vi "setPressure_topLvl.vi"(5 "which manipulator":T1(ring), 7 "Slide Refnum":refnum<vi>, 8 "error in":errorcluster, 10 "set pressure (mBar)":dbl format="%#_13g", 11 "Pressure box control in":T2={"Pressure box COM"="COM7", "pressure box type"=enum."Neuromatics", "High pos pressure (mBar)"=200.0, "Low pos pressure (mBar)"=80.0, "Vacuum pressure (mBar)"=-40.0, "calibration"=enum."mightenRig"}) -> (0 "error out":errorcluster, 3 "Pressure box control out":T2={"Pressure box COM"="", "pressure box type"=enum."Neuromatics", "High pos pressure (mBar)"=200.0, "Low pos pressure (mBar)"=80.0, "Vacuum pressure (mBar)"=-40.0, "calibration"=enum."PA_vacPump"})   [LabVIEW 2019]
uses:
  controls/pressure_box_control.ctl
  controls/pressure_box_type.ctl
  controls/arduino_pressure_setting.ctl
  controls/proportionAir_cmds.ctl
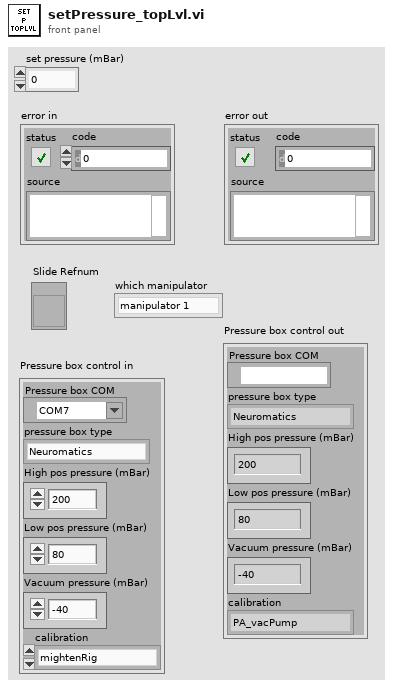
[diagram p1: front panel]
types:
  T1 = enum16{"manipulator 1", "manipulator 2", "manipulator 3", "manipulator 4"}
  T2 = typedef "pressure_box_control.ctl" = cluster{"Pressure box COM":refnum<visa-resource-name>, "pressure box type":T3, "High pos pressure (mBar)":dbl, "Low pos pressure (mBar)":dbl, "Vacuum pressure (mBar)":dbl, "calibration":enum16{"PA_vacPump", "PA_venturi", "Neuromatics", "ilyaRig", "mightenRig"}}
  T3 = typedef "pressure_box_type.ctl" = enum16{"Neuromatics", "ProportionAir", "Demo box", "N-ProportionAir"}
  T4 = enum16{"PA_vacPump", "PA_venturi", "Neuromatics", "ilyaRig", "mightenRig"}
  T5 = typedef "arduino_pressure_setting.ctl" = enum16{"High Positive Pressure", "Low Positive Pressure", "Atmospheric Pressure", "Low Vacuum", "High Vacuum", "Break In", "Puff"}
  T6 = typedef "proportionAir_cmds.ctl" = enum16{"Set P", "Switch to Atm", "Switch to Regulator", "Pulse", "WC"}
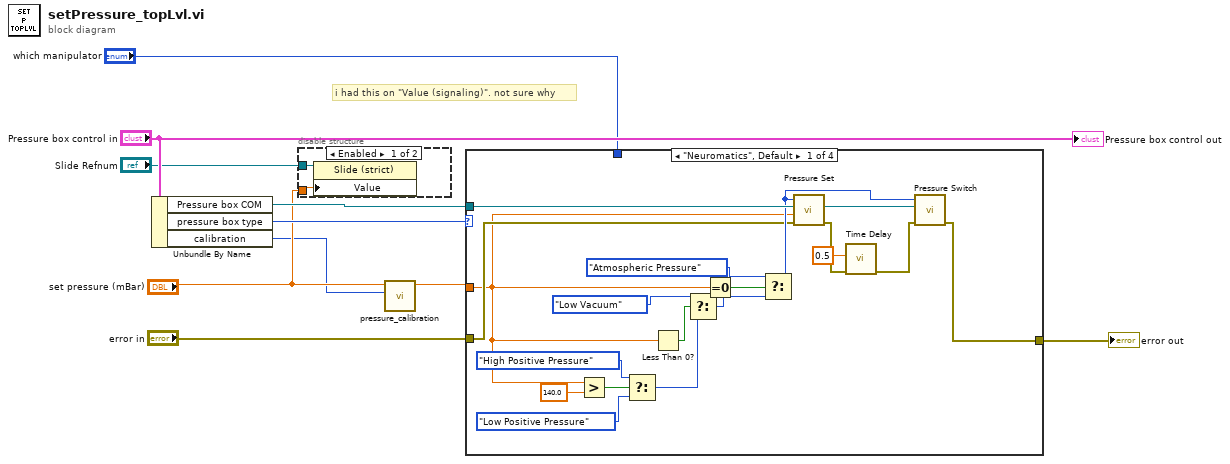
[diagram p0: block diagram]
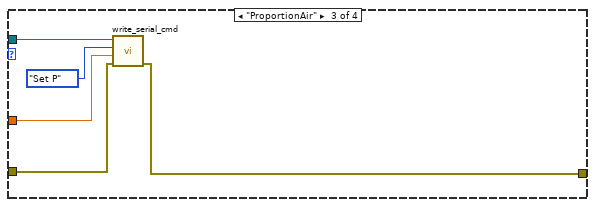
[diagram p4: hidden frame]
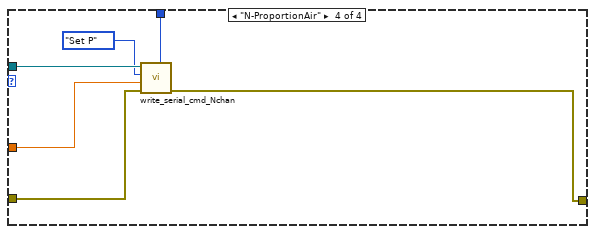
[diagram p5: hidden frame]
diagram:
  # "i had this on \"Value (signaling)\". not sure why"
  n1 = Unbundle By Name("Pressure box control in") -> ("Pressure box COM"=w9:refnum<visa-resource-name>, "pressure box type"=w10:T3, "calibration"=w1:T4)
  n2 = disable-structure shown="Enabled" {
    disable-tunnel: "Slide Refnum" -> [w12 _]
    disable-tunnel: "set pressure (mBar)" -> [w11 _]
    frame Enabled {
      n3 = property class="Slide (strict)"(reference=w12, "Value"=w11) -> ()  [unwired: 1 in, 2 out]
    }
    frame Disabled {
    }
  }
  n4 = call "pressure_calibration.vi"("calibration"=w1, "cmd pressure (mBar)"="set pressure (mBar)") -> ("pressure out (mbar)"=w5:dbl)  [unwired: 9 in]
  n5 = case shown="\"Neuromatics\", Default" w10 {
    tunnel: w9 -> [w27 _ w37 w43]
    tunnel: "error in" -> [w19 w32 w36 w39]
    tunnel: w5 -> [w18 _ w33 w40]
    tunnel: [w20 w32 w35 w38] -> w7
    tunnel: "which manipulator" -> [_ _ _ w41]
    frame "Neuromatics", Default {
      n6 = Greater?(x=w18, y=140.0) -> (0:w16:bool)
      n7 = Select(t=arduino_pressure_setting."High Positive Pressure" ("arduino pressure setting"), s=w16, f=arduino_pressure_setting."Low Positive Pressure" ("arduino pressure setting")) -> (s? t:f=w13:T5)
      n8 = Less Than 0?(x=w18) -> (x < 0?=w30:bool)
      n9 = Select(t=arduino_pressure_setting."Low Vacuum" ("arduino pressure setting"), s=w30, f=w13) -> (s? t:f=w31:T5)
      n10 = Equal To 0?(x=w18) -> (x = 0?=w25:bool)
      n11 = Select(t=arduino_pressure_setting."Atmospheric Pressure" ("arduino pressure setting"), s=w25, f=w31) -> (s? t:f=w22:T5)
      n12 = call "Pressure Set.vi"("error in"=w19, "Val"=w18, "Pressure Box COM"=w27, "arduino pressure setting"=w22) -> ("error out"=w24:errorcluster, "Pressure Box COM out"=w23:refnum<visa-resource-name>)  [unwired: 6 in]
      n13 = call "Time Delay"("error in (no error)"=w24, "Delay Time (s)"=0.5) -> ("error out"=w21:errorcluster)  [unwired: 9 in]
      n14 = call "Pressure Switch.vi"("error in"=w21, "Pressure Box COM"=w23, "arduino pressure setting"=w22) -> ("error out"=w20:errorcluster)  [unwired: 7 in, 1 out]
    }
    frame "Demo box" {
    }
    frame "ProportionAir" {
      n15 = call "write_serial_cmd.vi"("error in"=w36, "pressure set (mBar)"=w33, "pressure command"=proportionAir_cmds."Set P", "Pressure Box COM"=w37) -> ("error out"=w35:errorcluster)  [unwired: 6 in, 1 out]
    }
    frame "N-ProportionAir" {
      n16 = call "write_serial_cmd_Nchan.vi"("which manipulator"=w41, "error in"=w39, "arg 1"=w40, "pressure command"=proportionAir_cmds."Set P", "Pressure Box COM"=w43) -> ("error out"=w38:errorcluster)  [unwired: 5 in, 1 out]
    }
  }
  "error out" <- w7
  "Pressure box control out" <- "Pressure box control in"
